vi "Write Data.vi"(8 "error in (no error)":errorcluster, 10 "Data":string, 11 "Test Message in":refnum<class "Test Message.lvclass">) -> (0 "error out":errorcluster, 3 "Test Message out":refnum<class "Test Message.lvclass">)   [LabVIEW 2027, in "Test Message.lvclass"]
uses:
  Test Message.lvclass
  Test Message.lvclass/Test Message.ctl
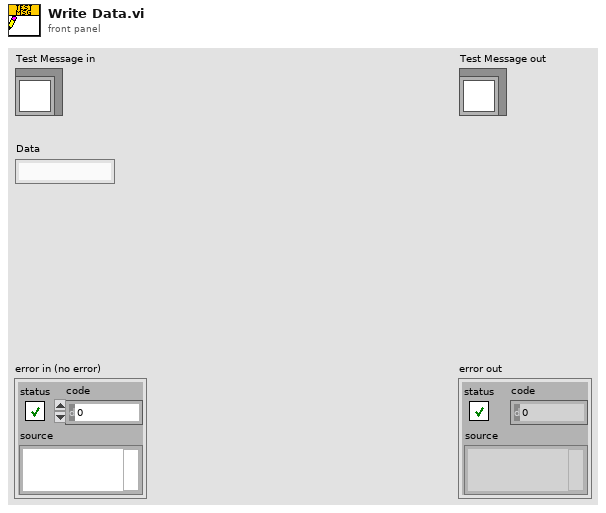
[diagram p1: front panel]
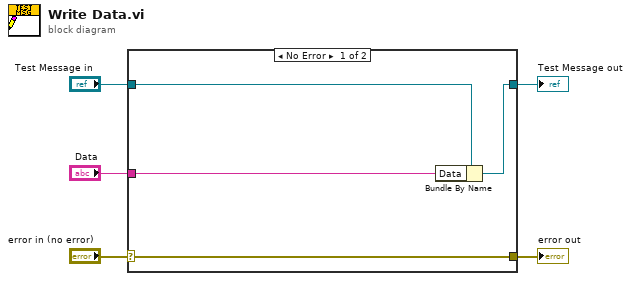
[diagram p0: block diagram]
diagram:
  n1 = case shown="No Error" "error in (no error)" {
    selector: "error in (no error)" -> [w9 w10]
    tunnel: [w9 w10] -> w4
    tunnel: [w7 w11] -> w2
    tunnel: "Test Message in" -> [w8 w11]
    tunnel: "Data" -> [w6 _]
    frame No Error {
      n2 = Bundle By Name(cluster=w8, "Data"=w6) -> (w7:refnum<class "Test Message.lvclass">)
    }
    frame Error {
    }
  }
  "error out" <- w4
  "Test Message out" <- w2
